vi "firstChildNode.vi"(8 "error in (no error)":errorcluster caption="errorIn", 11 "parentNode":refnum<k20>) -> (0 "error out":errorcluster caption="errorOut", 2 "found child node?":bool caption="found？", 3 "childNode":refnum<k20>)   [LabVIEW 2017]
uses:
  <vilib>/xml/Close Reference(Node).vi
  <vilib>/xml/NI_XML.lvlib
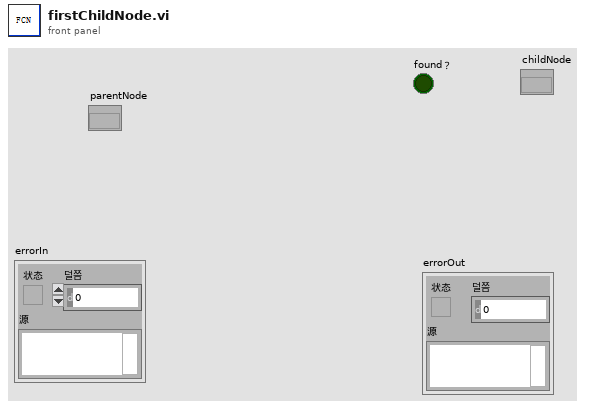
[diagram p1: front panel]
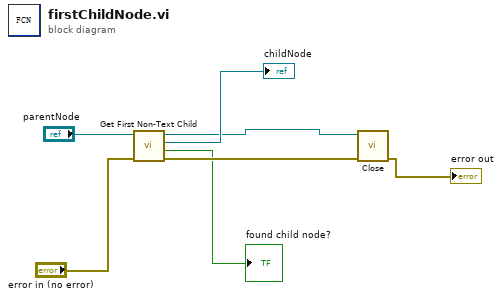
[diagram p0: block diagram]
diagram:
  n1 = call <vilib>:"Get First Non-Text Child.vi"("error in (no error)"="error in (no error)", "node in"="parentNode") -> ("error out"=w4:errorcluster, "found child node?"=→"found child node?":bool, "child node"=→"childNode":refnum<k20>, "node out"=w2:refnum<k20>)  [unwired: 6 out]
  n2 = call-poly <vilib>:"Close.vi"("error in (no error)"=w4, "node"=w2) -> ("error out"=→"error out":errorcluster)  [unwired: 7 in]
